vi "Read State.vi"(8 "error in (no error)":errorcluster, 11 "Channel GEI in":refnum<class "Channel.lvclass">) -> (0 "error out":errorcluster, 2 "State":string, 3 "Channel GEI out":refnum<class "Channel.lvclass">)   [LabVIEW 2018, in "Channel.lvclass"]
uses:
  Channel.lvclass
  Channel.lvclass/Channel.ctl
  State Machine/State Machine.lvclass
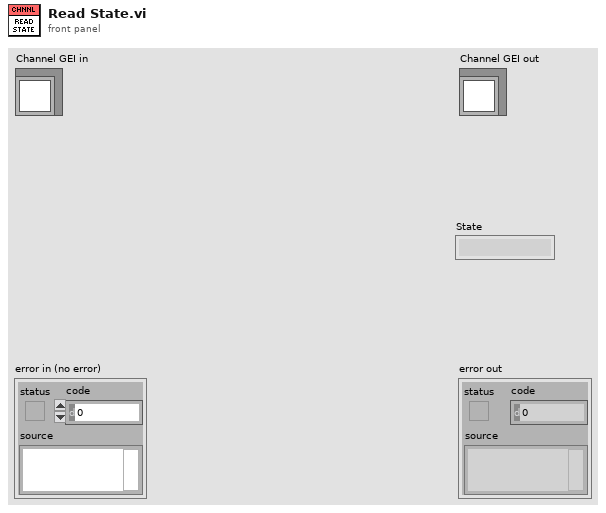
[diagram p1: front panel]
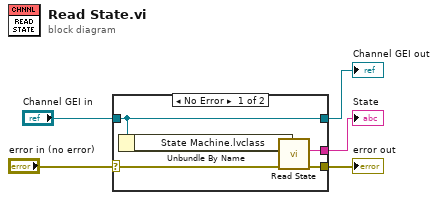
[diagram p0: block diagram]
diagram:
  n1 = case shown="No Error" "error in (no error)" {
    selector: "error in (no error)" -> [w8 w12]
    tunnel: [w6 w12] -> w4
    tunnel: [w10 w11] -> w2
    tunnel: "Channel GEI in" -> [w10 w11]
    tunnel: [w7 _] -> w1
    frame No Error {
      n2 = Unbundle By Name(w10) -> ("State Machine.lvclass"=w9:refnum<class "State Machine.lvclass">)
      n3 = call-dynamic "Read State.vi"("error in (no error)"=w8, "State Machine in"=w9) -> ("error out"=w6:errorcluster, "State"=w7:string)  [unwired: 7 in, 1 out]
    }
    frame Error {
    }
  }
  "error out" <- w4
  "Channel GEI out" <- w2
  "State" <- w1
